vi "Wordle.vi"(11 "Submission LLB":path) -> (0 "error out":errorcluster, 2 "Test Summary":string, 3 "Score":T1)   [LabVIEW 2020]
uses:
  Solver State.ctl
  Valid Guesses--constant.vi
  <vilib>/AdvancedString/Delimited String to 1D String Array.vi
panel:
  out "Current Solve":i32
  out "Elapsed Time":dbl
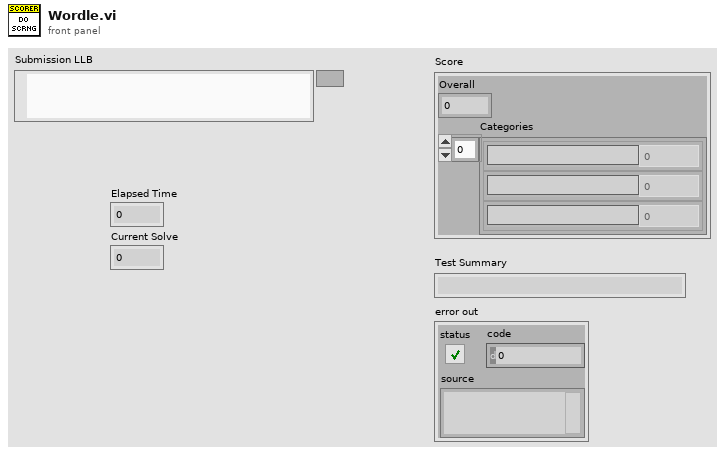
[diagram p1: front panel]
types:
  T1 = cluster{"Overall":dbl, "Categories":cluster{"Category":string, "Value":dbl}[]}
  T2 = typedef "Solver State.ctl" = enum16{"Init", "Test LLB", "Run", "Close"}
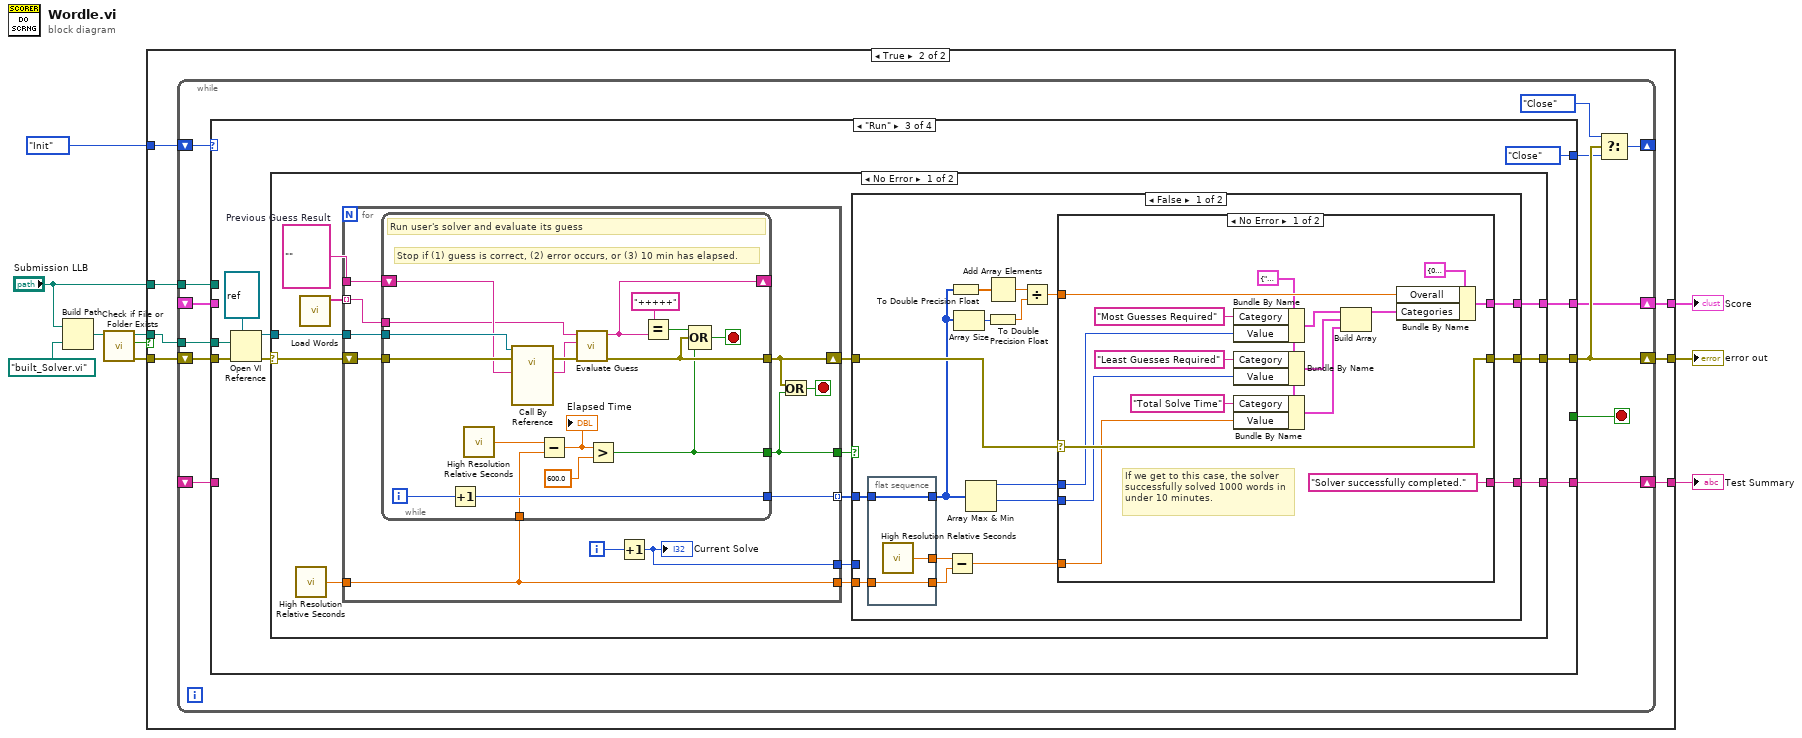
[diagram p0: block diagram]
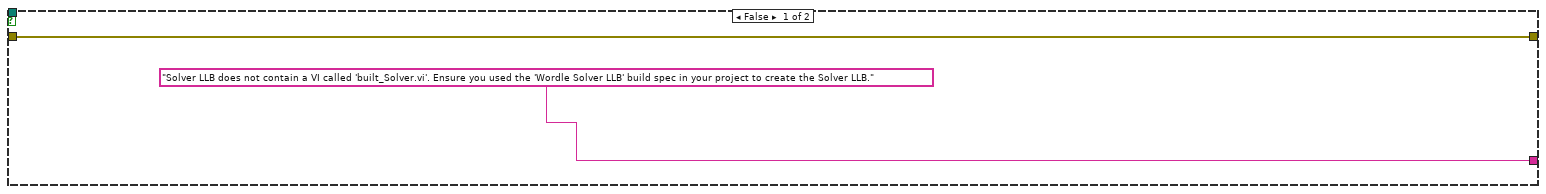
[diagram p2: hidden frame]
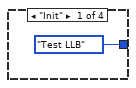
[diagram p3: hidden frame]
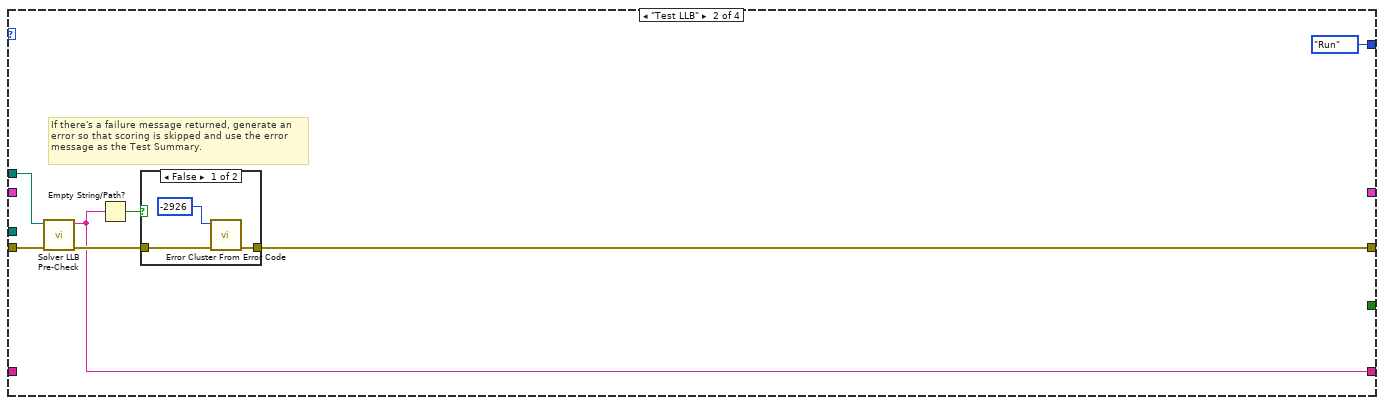
[diagram p4: hidden frame]
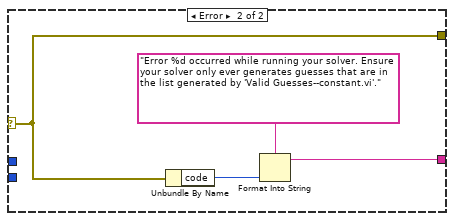
[diagram p6: hidden frame]
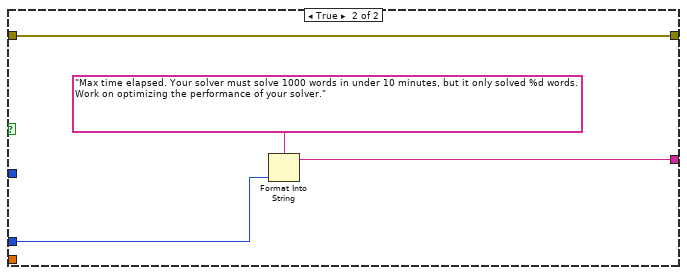
[diagram p7: hidden frame]
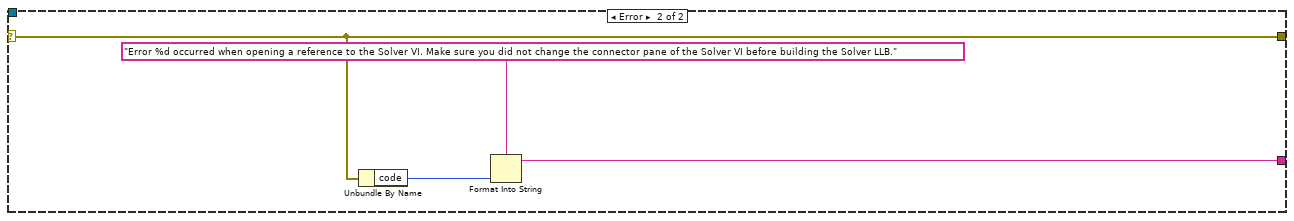
[diagram p8: hidden frame]
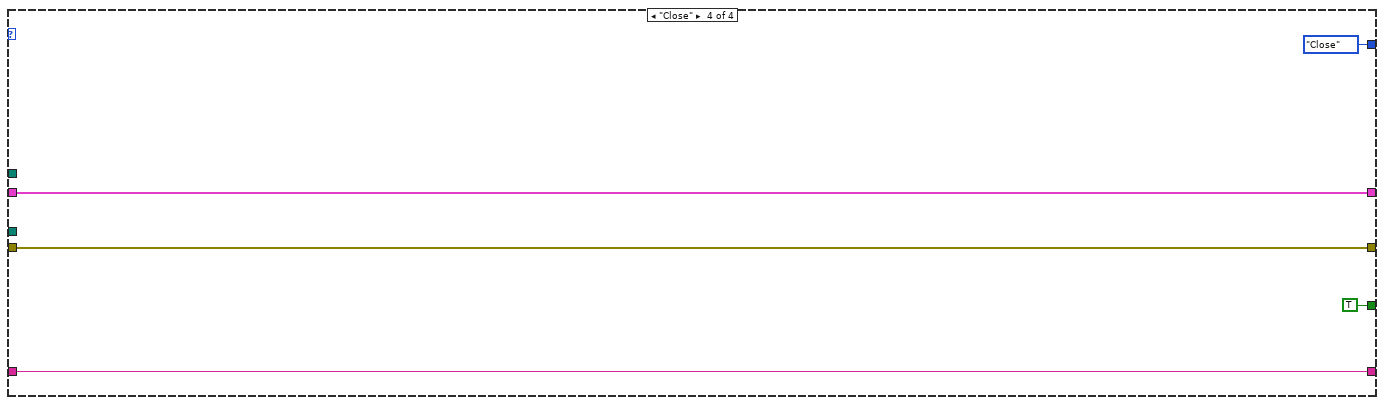
[diagram p9: hidden frame]
diagram:
  n1 = Build Path(base path="Submission LLB", name or relative path=path "built_Solver.vi") -> (appended path=w9:path)
  n2 = call <vilib>:"Check if File or Folder Exists.vi"("path"=w9) -> ("error out"=w5:errorcluster, "file or folder exists?"=w7:bool, "dup path"=w8:path)  [unwired: 8 in]
  n3 = case shown="True" w7 {
    tunnel: w8 -> [_ w18]
    tunnel: [w12 w17] -> w6
    tunnel: w5 -> [w12 w19]
    tunnel: ["Solver LLB does not contain a VI called 'built_Solver.vi'. Ensure you used the 'Wordle Solver LLB' build spec in your project to create the Solver LLB." w16] -> w4
    tunnel: [_ w15] -> w3
    tunnel: Solver_State."Init" ("Solver State") -> [_ w14]
    tunnel: "Submission LLB" -> [_ w13]
    frame False {
    }
    frame True {
      n4 = while {
        tunnel: w18 -> [w30]
        shift-right: [w32] -> w17
        shift-left: w19 -> [w31]
        shift-right: [w26] -> _
        shift-left: w14 -> [w27]
        shift-right: [w28] -> w15
        shift-left: _ -> [w23]
        shift-right: [w29] -> w16
        shift-left: _ -> [w22]
        tunnel: w13 -> [w20]
        stop <- w21 stop-if-true
        n5 = case shown="\"Run\"" w27 {
          tunnel: w31 -> [_ w39 w53 w147]
          tunnel: w30 -> [_ _ w52 _]
          tunnel: [_ w36 w49 w147] -> w32
          tunnel: [_ w35 w47 w146] -> w29
          tunnel: [_ _ w46 w148] -> w28
          tunnel: [Solver_State."Test LLB" ("Solver State") Solver_State."Run" ("Solver State") Solver_State."Close" ("Solver State") Solver_State."Close" ("Solver State")] -> w25
          tunnel: w23 -> [_ _ _ w148]
          tunnel: w22 -> [_ _ _ w146]
          tunnel: [_ _ _ TRUE] -> w21
          tunnel: w20 -> [_ w34 _ _]
          frame "Init" {
          }
          frame "Test LLB" {
            # "If there's a failure message returned, generate an error so that scoring is skipped and use the error message as the Test Summary."
            n6 = call "Solver LLB Pre-Check.vi"("error in"=w39, "Solver LLB"=w34) -> ("error out"=w38:errorcluster, "Issues Detected"=w35:string)  [unwired: 8 in]
            n7 = Empty String/Path?(string/path=w35) -> (empty?=w37:bool)
            n8 = case shown="False" w37 {
              tunnel: w38 -> [w43 w44]
              tunnel: [w42 w44] -> w36
              frame False {
                n9 = call <vilib>:"Error Cluster From Error Code.vi"("error in (no error)"=w43, "error code (0)"=-2926) -> ("error out"=w42:errorcluster)  [unwired: 7 in]
              }
              frame True {
              }
            }
          }
          frame "Run" {
            n10 = Open VI Reference(type specifier VI Refnum (for type only)=refnum<vi> refnum, vi path=w52, error in (no error)=w53) -> (vi reference=w48:refnum<vi>, error out=w50:errorcluster)  [unwired: 3 in]
            n11 = case shown="No Error" w50 {
              selector: w50 -> [w66 w140]
              tunnel: [w59 w140] -> w49
              tunnel: w48 -> [w65 _]
              tunnel: [w58 w142] -> w47
              tunnel: [w57 _] -> w46
              frame No Error {
                w64 = ""  # Previous Guess Result
                n12 = call <vilib>:"High Resolution Relative Seconds.vi"() -> ("relative seconds"=w63:dbl)
                n13 = call "Load Words.vi"() -> ("Words"=w54:string[])  [unwired: 11 in]
                n14 = for {
                  tunnel: w65 -> [w77]
                  shift-right: [w75] -> w60
                  shift-left: w66 -> [w76]
                  tunnel: w54 -> [w73] mode=indexing
                  tunnel: w64 -> [w72]
                  tunnel: [w71] -> w61 mode=indexing
                  tunnel: w63 -> [w70]
                  tunnel: [w70] -> w62
                  tunnel: [w68] -> w56
                  tunnel: [w67] -> w55
                  i -> [w74]
                  stop <- w69 stop-if-true
                  n15 = while {
                    tunnel: w77 -> [w95]
                    tunnel: w76 -> [w94]
                    tunnel: [w86] -> w75
                    shift-right: [w83] -> _
                    shift-left: w72 -> [w93]
                    tunnel: w73 -> [w85]
                    tunnel: [w88] -> w71
                    tunnel: w70 -> [w81]
                    tunnel: [w78] -> w68
                    i -> [w89]
                    stop <- w92 stop-if-true
                    # "Stop if (1) guess is correct, (2) error occurs, or (3) 10 min has elapsed."
                    # "Run user's solver and evaluate its guess"
                    n16 = Increment(x=w89) -> (x+1=w88:i32)
                    n17 = call <vilib>:"High Resolution Relative Seconds.vi"() -> ("relative seconds"=w82:dbl)
                    n18 = call-by-ref "?"(reference=w95, error in=w94, "Previous Guess Result"=w93) -> (error out=w87:errorcluster, "New Guess"=w84:string)  [unwired: 10 in, 1 out]
                    n19 = Subtract(x=w82, y=w81) -> (x-y=w80:dbl)
                    "Elapsed Time" <- w80
                    n20 = call "Evaluate Guess.vi"("error in"=w87, "Guess"=w84, "Current Word"=w85) -> ("error out"=w86:errorcluster, "Result"=w83:string)  [unwired: 7 in]
                    n21 = Greater?(x=w80, y=600.0) -> (0:w78:bool)
                    n22 = Equal?(x="+++++", y=w83) -> (x = y?=w90:bool)
                    n23 = Compound Arithmetic op=OR(w90, w86, w78) -> (w92:bool)
                  }
                  n24 = Increment(x=w74) -> (x+1=w67:i32)
                  "Current Solve" <- w67
                  n25 = Or(x=w75, y=w68) -> (x .or. y?=w69:bool)
                }
                n26 = case shown="False" w56 {
                  tunnel: w62 -> [w112 _]
                  tunnel: w61 -> [w102 _]
                  tunnel: w60 -> [w109 w139]
                  tunnel: [w108 w139] -> w59
                  tunnel: [w107 w136] -> w58
                  tunnel: [w106 _] -> w57
                  tunnel: w55 -> [_ w137]
                  frame False {
                    n27 = flat-sequence {
                      tunnel: [w135] -> w110
                      tunnel: w112 -> [w135]
                      tunnel: [w134] -> w111
                      tunnel: w102 -> [w133]
                      tunnel: [w133] -> w101
                      frame #0 {
                        n28 = call <vilib>:"High Resolution Relative Seconds.vi"() -> ("relative seconds"=w134:dbl)
                      }
                    }
                    n29 = Subtract(x=w111, y=w110) -> (x-y=w103:dbl)
                    n30 = To Double Precision Float(number=w101) -> (double precision float=w100:dbl[])
                    n31 = Array Size(array=w101) -> (size(s)=w98:i32)
                    n32 = Array Max & Min(array=w101) -> (max value=w105:i32, min value=w104:i32)  [unwired: 2 out]
                    n33 = Add Array Elements(numeric array=w100) -> (sum=w99:dbl)
                    n34 = To Double Precision Float(number=w98) -> (double precision float=w97:dbl)
                    n35 = Divide(x=w99, y=w97) -> (x/y=w96:dbl)
                    n36 = case shown="No Error" w109 {
                      selector: w109 -> [w128 w129]
                      tunnel: [w128 w129] -> w108
                      tunnel: ["Solver successfully completed." w131] -> w107
                      tunnel: [w125 _] -> w106
                      tunnel: w96 -> [w124 _]
                      tunnel: w105 -> [w121 _]
                      tunnel: w104 -> [w118 _]
                      tunnel: w103 -> [w113 _]
                      frame No Error {
                        w114 = cluster{"Category":string, "Value":dbl} {"Category"="", "Value"=0.0} ("Score Entry")
                        # "If we get to this case, the solver successfully solved 1000 words in under 10 minutes."
                        n37 = Bundle By Name(cluster=w114, "Category"="Most Guesses Required", "Value"=w121) -> (w119:cluster{"Category":string, "Value":dbl})
                        n38 = Bundle By Name(cluster=w114, "Category"="Least Guesses Required", "Value"=w118) -> (w117:cluster{"Category":string, "Value":dbl})
                        n39 = Bundle By Name(cluster=w114, "Category"="Total Solve Time", "Value"=w113) -> (w115:cluster{"Category":string, "Value":dbl})
                        n40 = Build Array(w119, w117, w115) -> (w123:cluster{"Category":string, "Value":dbl}[])
                        n41 = Bundle By Name(cluster=T1 {"Overall"=0.0, "Categories"=[]} ("Score"), "Overall"=w124, "Categories"=w123) -> (w125:T1)
                      }
                      frame Error {
                        n42 = Unbundle By Name(w129) -> ("code"=w130:i32)
                        n43 = Format Into String(format string="Error %d occurred while running your solver. Ensure your solver only ever generates guesses that are in the list generated by 'Valid Guesses--constant.vi'.", w130) -> (resulting string=w131:string)  [unwired: 2 in, 1 out]
                      }
                    }
                  }
                  frame True {
                    n44 = Format Into String(format string="Max time elapsed. Your solver must solve 1000 words in under 10 minutes, but it only solved %d words. Work on optimizing the performance of your solver.", w137) -> (resulting string=w136:string)  [unwired: 2 in, 1 out]
                  }
                }
              }
              frame Error {
                n45 = Unbundle By Name(w140) -> ("code"=w141:i32)
                n46 = Format Into String(format string="Error %d occurred when opening a reference to the Solver VI. Make sure you did not change the connector pane of the Solver VI before building the Solver LLB.", w141) -> (resulting string=w142:string)  [unwired: 2 in, 1 out]
              }
            }
          }
          frame "Close" {
          }
        }
        n47 = Select(t=Solver_State."Close", s=w32, f=w25) -> (s? t:f=w26:T2)
      }
    }
  }
  "Score" <- w3
  "Test Summary" <- w4
  "error out" <- w6
